vi "Obtain Queue.vi"(2 "error in":errorcluster, 3 "data type":variant, 4 "Queue":T1) -> (0 "error out":errorcluster, 1 "Queue Ref":refnum<queue>)   [LabVIEW 2016]
uses:
  Refname/Queues.ctl
  Refname/Refname to String (Queues).vi
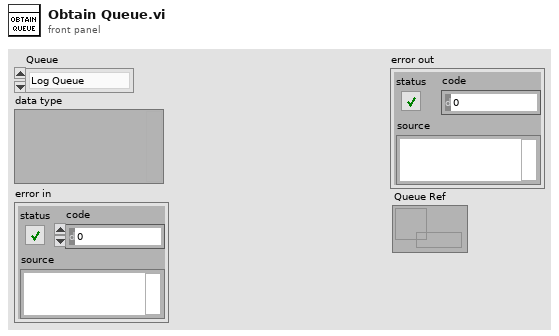
[diagram p1: front panel]
types:
  T1 = typedef "Queues.ctl" = enum16{"Log Queue"}
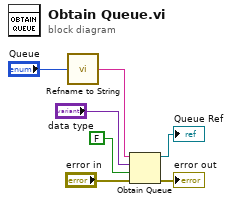
[diagram p0: block diagram]
diagram:
  n1 = call-poly "Refname to String.vi"("Enum"="Queue") -> ("String"=w6:string)
  n2 = Obtain Queue(name (unnamed)=w6, element data type="data type", create if not found? (T)=FALSE, error in (no error)="error in") -> (queue out=→"Queue Ref":refnum<queue>, error out=→"error out":errorcluster)  [unwired: 1 in, 1 out]
